vi "Move.vi"(8 "error in (no error)":errorcluster, 11 "StageSPIM in":refnum<class "StageSPIM.lvclass">) -> (0 "error out":errorcluster, 3 "StageSPIM out":refnum<class "StageSPIM.lvclass">)   [LabVIEW 2012, in "StageSPIM.lvclass"]
uses:
  StageSPIM.lvclass
  StageSPIM.lvclass/StageSPIM.ctl
panel:
  out "Target position":dbl[][](array[numeric])
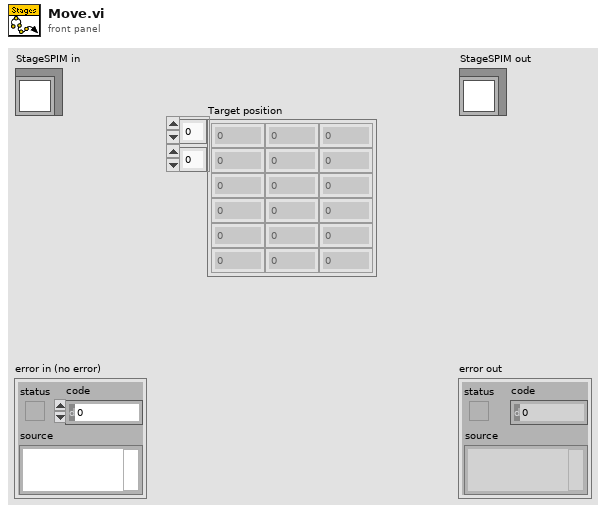
[diagram p1: front panel]
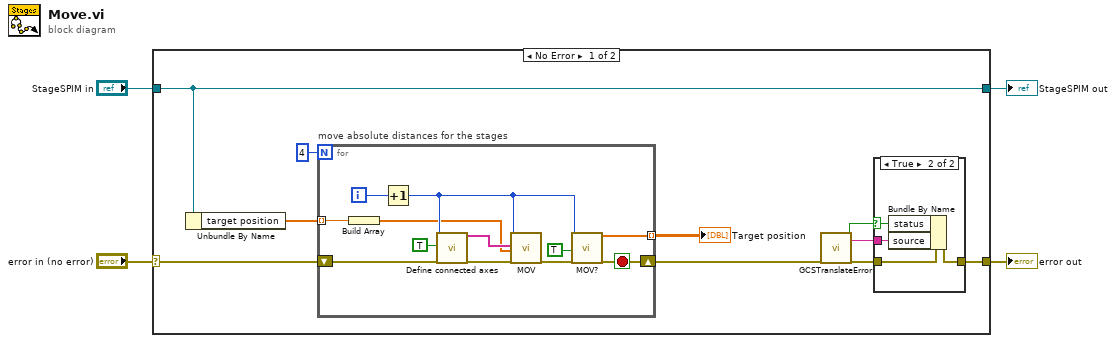
[diagram p0: block diagram]
diagram:
  n1 = case shown="No Error" "error in (no error)" {
    selector: "error in (no error)" -> [w13 w33]
    tunnel: [w9 w33] -> w3
    tunnel: [w12 w32] -> w1
    tunnel: "StageSPIM in" -> [w12 w32]
    frame No Error {
      n2 = Unbundle By Name(w12) -> ("target position"=w11:dbl[])
      n3 = for "move absolute distances for the stages" {
        N: 4 -> [_]
        shift-right: [w21] -> w5
        shift-left: w13 -> [w30]
        tunnel: w11 -> [w31] mode=indexing
        tunnel: [w20] -> w6 mode=indexing
        i -> [w29]
        stop <- w21 stop-if-true
        n4 = Build Array(w31) -> (w23:dbl[])
        n5 = Increment(x=w29) -> (x+1=w28:i32)
        n6 = call "Define connected axes.vi"("System no."=w28, "Read from\ncontroller?"=TRUE ("Read from\ncontroller?"), "error in"=w30) -> ("Conn. Axes out"=w24:string[], "error out"=w27:errorcluster)  [unwired: 15 in]
        n7 = call "MOV.vi"("System no."=w28, "Axes to move"=w24, "Position values"=w23, "error in"=w27) -> ("error out"=w26:errorcluster)  [unwired: 15 in]
        n8 = call "MOV?.vi"("System no."=w28, "All axes?"=TRUE, "error in"=w26) -> ("Target position"=w20:dbl[], "error out"=w21:errorcluster)  [unwired: 15 in]
      }
      "Target position" <- w6
      n9 = call "GCSTranslateError.vi"("error in"=w5) -> ("GCS Error?"=w8:bool, "Error Description"=w7:string, "error out"=w10:errorcluster)  [unwired: 16 in]
      n10 = case shown="True" w8 {
        selector: w8 -> [_ w17]
        tunnel: w10 -> [w15 w19]
        tunnel: [w15 w18] -> w9
        tunnel: w7 -> [_ w16]
        frame False {
        }
        frame True {
          n11 = Bundle By Name(cluster=w19, "status"=w17, "source"=w16) -> (w18:errorcluster)
        }
      }
    }
    frame Error {
    }
  }
  "error out" <- w3
  "StageSPIM out" <- w1
